vi "numCmd_Send_Generic.vi"(7 "Command Name":string, 11 "Value":variant) -> (0 "error out":errorcluster)   [LabVIEW 2019, in "Trajectory_Library.lvlib"]
uses:
  Trajectory_Library.lvlib
  numCmd_ObtainQueue.vi
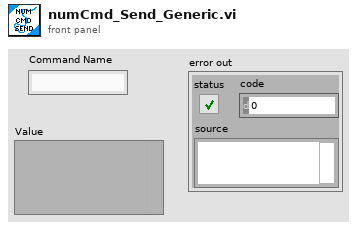
[diagram p1: front panel]
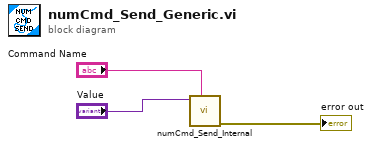
[diagram p0: block diagram]
diagram:
  n1 = call "numCmd_Send_Internal.vi"("Command Name"="Command Name", "Value"="Value") -> ("error out"=→"error out":errorcluster)  [unwired: 9 in]
